vi "Get Lat_Lon_TZ.vi"(8 "error in (no error)":errorcluster, 11 "API Output":string) -> (0 "error out":errorcluster, 2 "Lat, Long, Timezone":T1, 3 "API Output (copy)":string)   [LabVIEW 2017, in "Dark Sky Weather Data for LabVIEW.lvlib"]
doc: "Parses the Dark Sky API's output for latitude, longitude, and timezone info"
uses:
  Dark Sky Weather Data for LabVIEW.lvlib
  Controls/Lat_Lon_TZ.ctl
  <vilib>/addons/_JKI.lib/Serialization/JSON/JKI JSON Serialization.lvlib
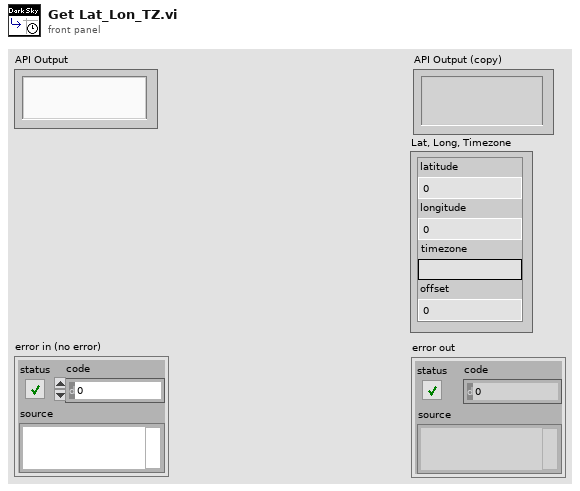
[diagram p1: front panel]
types:
  T1 = typedef "Dark Sky Weather Data for LabVIEW.lvlib/Lat_Lon_TZ.ctl" = cluster{"latitude":dbl, "longitude":dbl, "timezone":string, "offset":dbl}
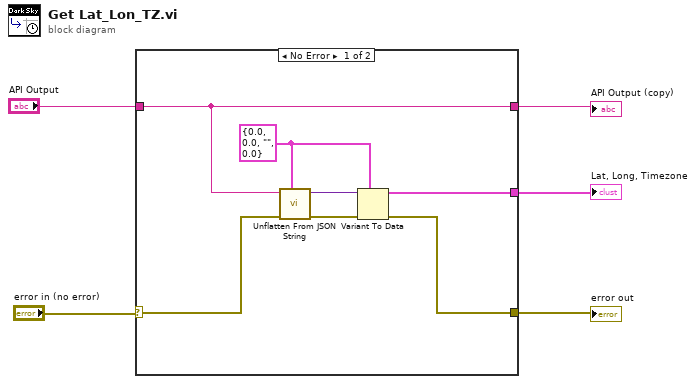
[diagram p0: block diagram]
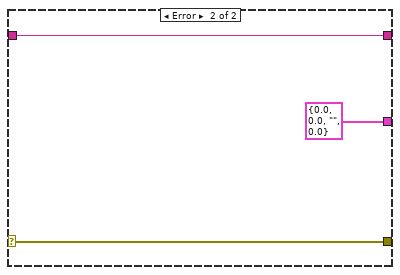
[diagram p2: hidden frame]
diagram:
  n1 = case shown="No Error" "error in (no error)" {
    selector: "error in (no error)" -> [w12 w15]
    tunnel: [w9 w15] -> w4
    tunnel: "API Output" -> [w6 w13]
    tunnel: [w7 T1 {"latitude"=0.0, "longitude"=0.0, "timezone"="", "offset"=0.0} ("Lat, Long, Timezone")] -> w2
    tunnel: [w6 w13] -> w1
    frame No Error {
      w8 = T1 {"latitude"=0.0, "longitude"=0.0, "timezone"="", "offset"=0.0} ("Lat, Long, Timezone")
      n2 = call <vilib>:"Unflatten From JSON String.vi"("Type and Defaults"=w8, "error in (no error)"=w12, "JSON String"=w6) -> ("error out"=w10:errorcluster, "Variant"=w11:variant)  [unwired: 7 in]
      n3 = Variant To Data(error in=w10, type=w8, Variant=w11) -> (data=w7:T1, error out=w9:errorcluster)
    }
    frame Error {
    }
  }
  "error out" <- w4
  "Lat, Long, Timezone" <- w2
  "API Output (copy)" <- w1
